vi "StartWebcam.vi"(6 "ResetWebcam?":bool=TRUE, 7 "NumWebcamImages":i32=1, 8 "WebcamOccurrence":refnum<k4>, 9 "Teleop?":bool=TRUE, 10 "WebcamStartTime (ms)":i32, 11 "ElapsedTime (ms)":i32) -> (2 "WebcamImagesProcessed":i32)   [LabVIEW 2013]
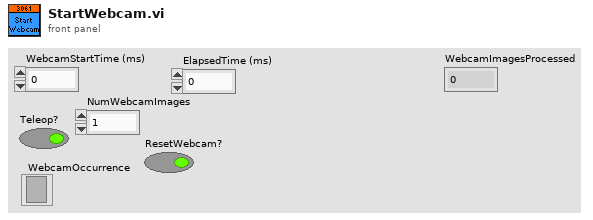
[diagram p1: front panel]
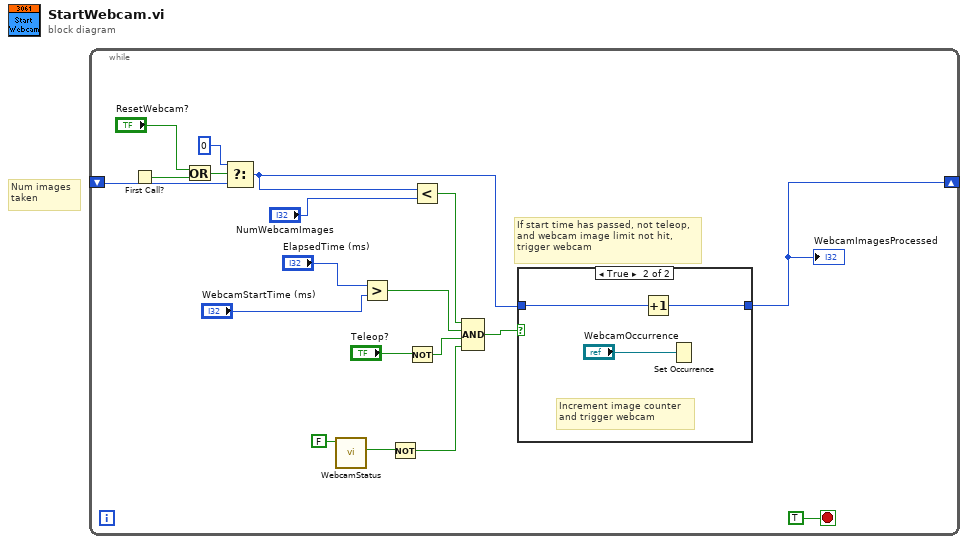
[diagram p0: block diagram]
diagram:
  # "Num images\ntaken"
  n1 = while {
    shift-right: [w7] -> _
    shift-left: _ -> [w9]
    stop <- TRUE stop-if-true
    # "If start time has passed, not teleop,\nand webcam image limit not hit,\ntrigger webcam"
    n2 = First Call?() -> (First Call?: T/F=w4:bool)
    n3 = Or(x="ResetWebcam?", y=w4) -> (x .or. y?=w6:bool)
    n4 = Select(t=0, s=w6, f=w9) -> (s? t:f=w8:i32)
    n5 = call "WebcamStatus.vi"("Write?"=FALSE) -> ("CurrentValue"=w2:bool)  [unwired: 10 in]
    n6 = Greater?(x="ElapsedTime (ms)", y="WebcamStartTime (ms)") -> (0:w13:bool)
    n7 = Not(x=w2) -> (.not. x?=w1:bool)
    n8 = Not(x="Teleop?") -> (.not. x?=w14:bool)
    n9 = Less?(x=w8, y="NumWebcamImages") -> (x < y?=w12:bool)
    n10 = Compound Arithmetic op=AND(w12, w13, w14, w1) -> (w11:bool)
    n11 = case shown="True" w11 {
      tunnel: w8 -> [w20 w22]
      tunnel: [w20 w21] -> w7
      frame False {
      }
      frame True {
        # "Increment image counter\nand trigger webcam"
        n12 = Increment(x=w22) -> (x+1=w21:i32)
        n13 = Set Occurrence("WebcamOccurrence") -> ()
      }
    }
    "WebcamImagesProcessed" <- w7
  }
